vi "ACT_Loop.vi"() -> ()   [LabVIEW 2023, in "Lift_ACT.lvlib"]
uses:
  Lift_ACT.lvlib
  RoboRIO Utilities/Global_STOP.vi
  ENUM_ACT_Action.ctl
  ENUM_ACT_State.ctl
  Global_CMD_ACT_Data In.vi
  Global_ACT_Data Out.vi
  Cluster_CMD_ACT_Data.ctl
  <vilib>/Rock Robotics/WPI/MotorControl/WPI_MotorControlType.ctl
  <vilib>/Rock Robotics/SystemInterfaces/DIO/FPGA_DIOPWMChannel.ctl
  <vilib>/Rock Robotics/WPI/PWM/WPI_PWMDeadband.ctl
  <vilib>/Rock Robotics/SystemInterfaces/DIO/FPGA_DIOChannel.ctl
  <vilib>/Rock Robotics/WPI/MotorControl/WPI_MotorControlDeviceRef.ctl
  <vilib>/Rock Robotics/WPI/ThirdParty/Phoenix-LabVIEW/Motor Controller/Controls/CTRE_Phoenix_MotorControl_TalonFXInvertType.ctl
  <vilib>/Rock Robotics/WPI/ThirdParty/Phoenix-LabVIEW/Motor Controller/Controls/CTRE_Phoenix_MotorControl_NeutralMode.ctl
  Shared Code/TypeDefs/Cluster_FWD  REV Values.ctl
  Shared Code/TypeDefs/Cluster_Config Motor Output.ctl
  Shared Code/TypeDefs/Cluster_PID Gains.ctl
  Shared Code/TypeDefs/Cluster_High-Low.ctl
  Shared Code/TypeDefs/Cluster_PID Config.ctl
  Shared Code/TypeDefs/Cluster_Motion Magic Parameters.ctl
  <vilib>/Rock Robotics/WPI/ThirdParty/Phoenix-LabVIEW/Motor Controller/Controls/CTRE_Phoenix_MotorControl_LimitSwitchNormal.ctl
  Shared Code/TypeDefs/Cluser_Hard Limits.ctl
  Shared Code/TypeDefs/Cluser_Enable-Value I32.ctl
  Shared Code/TypeDefs/Cluser_Config_Soft Limits.ctl
  Shared Code/TypeDefs/Cluser_Limit Travel Config.ctl
  b5508d6c-c1cc-4273-80c5-2077d34e1483.vi
  5f725c2a-0ce1-4524-8967-e83b15fdce90.vi
  <vilib>/Rock Robotics/WPI/ThirdParty/Phoenix-LabVIEW/Motor Controller/Controls/CTRE_Phoenix_MotorControl_ControlMode.ctl
  Shared Code/TypeDefs/Cluster_FX CloseLoop Values.ctl
  Shared Code/TypeDefs/Cluster_FX Limit Switchs.ctl
  Shared Code/TypeDefs/Cluster_FX Current Values.ctl
  Shared Code/TypeDefs/Cluster_Config_Cancoder Data.ctl
  <vilib>/Rock Robotics/WPI/ThirdParty/Phoenix-LabVIEW/CANCoder/Controls/CTRE_Phoenix_CANcoder_DeviceRef.ctl
  Shared Code/TypeDefs/Cluster_FX Sensor Values.ctl
  4f1f8321-3dc8-4b28-8619-20673fc77ec2.vi
  36677ea0-a1a5-47a3-bc56-4475cb7c281e.vi
  573e44c0-11f4-4bd9-ad56-904ec25dba75.vi
  e7494af9-f670-4352-9dfa-ae6ce50709ea.vi
  6201c2b1-dcd8-4430-86f1-9b4ee56c7753.vi
  Shared Code/TypeDefs/Cluster_Lift_Config HW Values.ctl
  Shared Code/TypeDefs/Cluster_Lift_Config SW Values.ctl
  Shared Code/TypeDefs/Cluster_Lift_HW Outputs.ctl
  Shared Code/TypeDefs/Cluster_Lift_SW Output Data.ctl
  5a6858c7-91b3-4b8f-b750-ef97bd4cf642.vi
  89a2f430-b809-46a3-beae-127ce7f74435.vi
  <vilib>/Rock Robotics/WPI/ThirdParty/Phoenix-LabVIEW/CANCoder/Get/CTRE_Phoenix_CANcoder_GetSensorData.vi
  Shared Code/TypeDefs/Cluster_FX Integrated Sensor Values.ctl
  Shared Code/TypeDefs/ENUM_Lift_CMD_Mode Select.ctl
  Shared Code/TypeDefs/Cluser_CAN Follower Data.ctl
  Shared Code/TypeDefs/Cluser_Config_Current Limits.ctl
panel:
  in  "CMD Override":enum32{"None", "Velocity", "Position", "STOP"}(tab)
  in  "Velocity":dbl(slide) scale=-0.2..0.2
  in  "Target Counts":i32
  in  "Positon GO":bool
  out "Current Time":timestamp
  in  "SW Config":T1={"LiftSW Ver"=0, "At Position Delay(S)"=0.2}
  out "SW Output":T2
  in  "Reset zero Offset on Limit Switch":bool
  out "Sensor Read time":dbl format="%.3f"
  out "HW Outputs":T3
  in  "Read Saved Config":bool
  in  "Update Config":bool
  in  "HW Config":T9={"LiftHW Ver"=0, "CAN"={"ID Primary"=0, "Bus"="", "ID Follower"=0}, "Output"={"Type"=enum."Counter-Clockwise", "Neutral"=enum."EEPROMSetting", "Max"={"FWD"=0.0, "REV"=0.0}, "Min"={"FWD"=0.0, "REV"=0.0}, "OL Ramp Rate (S)"=0.0, "Dead Band"=0.0}, "CLUp"={"Gains"={"P"=0.0, "I"=0.0, "D"=0.0, "F"=0.0}, "Error Allowed"={"High"=0.0, "Low"=0.0}, "I Zone"={"High"=0.0, "Low"=0.0}, "Max Out"={"FWD"=0.0, "REV"=0.0}, "Max I Accu"={"High"=0.0, "Low"=0.0}, "CL Ramp Rate (S)"=0.0}, "MM"={"Cruise Velocity"=0, "Acceleration"=0}, "TravelLimits"={"Hard"={"FWD Switch Normal"=enum."Normally Open", "FWD On will Zero Encoder "=FALSE, "REV Switch Normal"=enum."Normally Open", "REV On will Zero Encoder "=FALSE}, "Soft"={"FWD"={"Enable"=FALSE, "Counts"=0}, "REV"={"Enable"=FALSE, "Counts"=0}}}, "Cancoder"={"ID"=0, "CW(t) CCW(f)"=TRUE, "Zero Offset"=0.0}, "CLDown"={"Gains"={"P"=1.0, "I"=0.01, "D"=0.0, "F"=0.0}, "Error Allowed"={"High"=0.0, "Low"=0.0}, "I Zone"={"High"=10000.0, "Low"=-1000.0}, "Max Out"={"FWD"=1.0, "REV"=-1.0}, "Max I Accu"={"High"=10.0, "Low"=-10.0}, "CL Ramp Rate (S)"=0.0}, "CurrentLimit"={"Enable"=FALSE, "Current Limit"=0.0, "Threshold Current"=0.0, "Threshold Time"=0.0}} {"CLDown"."Max I Accu"."Low" format="%#.8f"; "CLDown"."Max I Accu"."High" format="%#.8f"; "CLDown"."Gains"."F" format="%#.8f"; "CLDown"."Gains"."D" format="%#.8f"; "CLDown"."Gains"."I" format="%#.8f"; "CLDown"."Gains"."P" format="%#.8f"; "CLDown"."Error Allowed"."Low" format="%#.8f"; "CLDown"."Error Allowed"."High" format="%#.8f"; "CLDown"."I Zone"."Low" format="%#.8f"; "CLDown"."I Zone"."High" format="%#.8f"; "CLDown"."Max Out"."REV" format="%.2f"; "CLDown"."Max Out"."FWD" format="%.2f"; "TravelLimits"."Soft"."REV"."Counts" format="%#.0f"; "TravelLimits"."Soft"."FWD"."Counts" format="%#.0f"; "Output"."Min"."REV" format="%.2f"; "Output"."Min"."FWD" format="%.2f"; "Output"."Max"."REV" format="%.2f"; "Output"."Max"."FWD" format="%.2f"; "CLUp"."Max I Accu"."Low" format="%#.8f"; "CLUp"."Max I Accu"."High" format="%#.8f"; "CLUp"."Gains"."F" format="%#.8f"; "CLUp"."Gains"."D" format="%#.8f"; "CLUp"."Gains"."I" format="%#.8f"; "CLUp"."Gains"."P" format="%#.8f"; "CLUp"."Error Allowed"."Low" format="%#.8f"; "CLUp"."Error Allowed"."High" format="%#.8f"; "CLUp"."I Zone"."Low" format="%#.8f"; "CLUp"."I Zone"."High" format="%#.8f"; "CLUp"."Max Out"."REV" format="%.2f"; "CLUp"."Max Out"."FWD" format="%.2f"}
  out "CMD":T26
  out "Cycle Time (S)":dbl format="%.3g"
  # "STOP"
  # "Tune Output\nto 1023 Max"
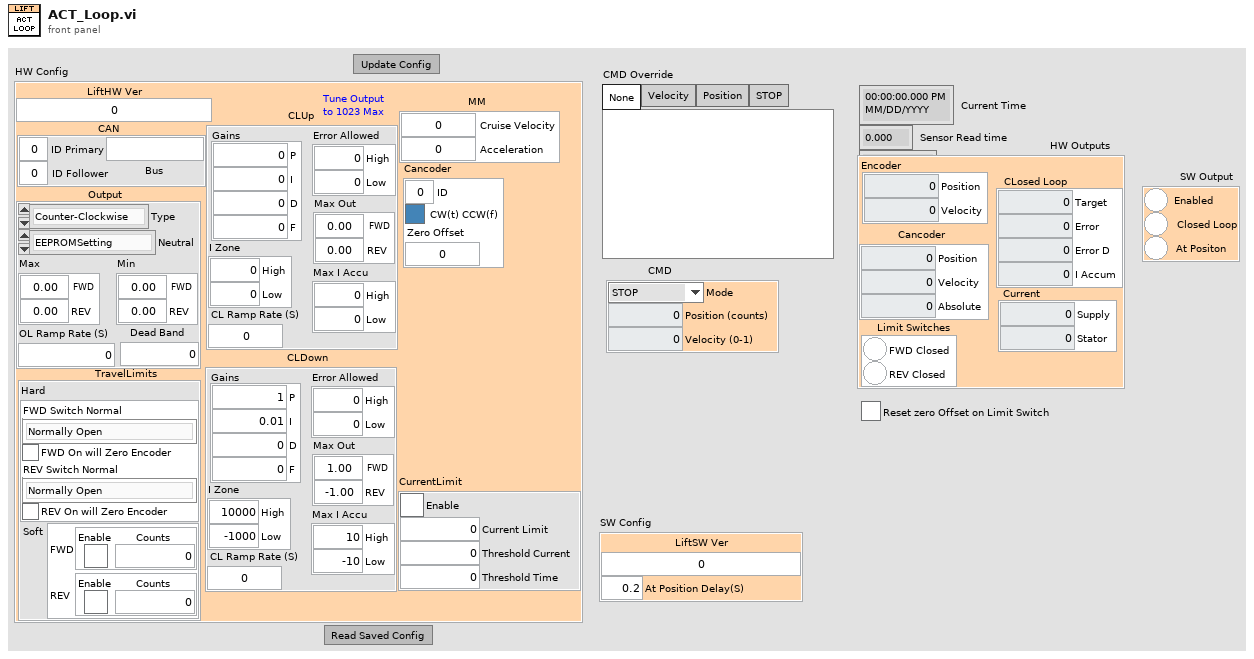
[diagram p1: front panel]
types:
  T1 = typedef "Cluster_Lift_Config SW Values.ctl" = cluster{"LiftSW Ver":u64, "At Position Delay(S)":dbl}
  T2 = typedef "Cluster_Lift_SW Output Data.ctl" = cluster{"Enabled":bool, "Closed Loop":bool, "At Positon":bool}
  T3 = typedef "Cluster_Lift_HW Outputs.ctl" = cluster{"Encoder":T4, "CLosed Loop":T5, "Limit Switches":T6, "Current":T7, "Cancoder":T8}
  T4 = typedef "Cluster_FX Sensor Values.ctl" = cluster{"Position":i32, "Velocity":i32}
  T5 = typedef "Cluster_FX CloseLoop Values.ctl" = cluster{"Target":dbl, "Error":i32, "Error D":dbl, "I Accum":dbl}
  T6 = typedef "Cluster_FX Limit Switchs.ctl" = cluster{"FWD Closed":bool, "REV Closed":bool}
  T7 = typedef "Cluster_FX Current Values.ctl" = cluster{"Supply":dbl, "Stator":dbl}
  T8 = typedef "Cluster_FX Integrated Sensor Values.ctl" = cluster{"Position":dbl, "Velocity":dbl, "Absolute":dbl}
  T9 = typedef "Cluster_Lift_Config HW Values.ctl" = cluster{"LiftHW Ver":u64, "CAN":T10, "Output":T11, "CLUp":T15, "MM":T18, "TravelLimits":T19, "Cancoder":T24, "CLDown":T15, "CurrentLimit":T25}
  T10 = typedef "Cluser_CAN Follower Data.ctl" = cluster{"ID Primary":u8, "Bus":string, "ID Follower":u8}
  T11 = typedef "Cluster_Config Motor Output.ctl" = cluster{"Type":T12, "Neutral":T13, "Max":T14, "Min":T14, "OL Ramp Rate (S)":dbl, "Dead Band":dbl}
  T12 = typedef "CTRE_Phoenix_MotorControl_TalonFXInvertType.ctl" = enum16{"Counter-Clockwise", "Clockwise"}
  T13 = typedef "CTRE_Phoenix_MotorControl_NeutralMode.ctl" = enum8{"EEPROMSetting", "Override to Coast", "Override to Brake"}
  T14 = typedef "Cluster_FWD  REV Values.ctl" = cluster{"FWD":dbl, "REV":dbl}
  T15 = typedef "Cluster_PID Config.ctl" = cluster{"Gains":T16, "Error Allowed":T17, "I Zone":T17, "Max Out":T14, "Max I Accu":T17, "CL Ramp Rate (S)":dbl}
  T16 = typedef "Cluster_PID Gains.ctl" = cluster{"P":dbl, "I":dbl, "D":dbl, "F":dbl}
  T17 = typedef "Cluster_High-Low.ctl" = cluster{"High":dbl, "Low":dbl}
  T18 = typedef "Cluster_Motion Magic Parameters.ctl" = cluster{"Cruise Velocity":i32, "Acceleration":i32}
  T19 = typedef "Cluser_Limit Travel Config.ctl" = cluster{"Hard":T20, "Soft":T22}
  T20 = typedef "Cluser_Hard Limits.ctl" = cluster{"FWD Switch Normal":T21, "FWD On will Zero Encoder ":bool, "REV Switch Normal":T21, "REV On will Zero Encoder ":bool}
  T21 = typedef "CTRE_Phoenix_MotorControl_LimitSwitchNormal.ctl" = enum16{"Normally Open", "Normally Closed", "Disabled"}
  T22 = typedef "Cluser_Config_Soft Limits.ctl" = cluster{"FWD":T23, "REV":T23}
  T23 = typedef "Cluser_Enable-Value I32.ctl" = cluster{"Enable":bool, "Counts":i32}
  T24 = typedef "Cluster_Config_Cancoder Data.ctl" = cluster{"ID":u8, "CW(t) CCW(f)":bool, "Zero Offset":dbl}
  T25 = typedef "Cluser_Config_Current Limits.ctl" = cluster{"Enable":bool, "Current Limit":dbl, "Threshold Current":dbl, "Threshold Time":dbl}
  T26 = typedef "Lift_ACT.lvlib/Cluster_CMD_ACT_Data.ctl" = cluster{"Mode":T27, "Position (counts)":i32, "Velocity (0-1)":dbl}
  T27 = typedef "ENUM_Lift_CMD_Mode Select.ctl" = enum16{"STOP", "Position", "Percent out"}
  T28 = typedef "CTRE_Phoenix_CANcoder_DeviceRef.ctl" = cluster{"DeviceStatus":errorcluster, "Device Number":u8, "Handle":u64, "UsageFrame":u32, "Library Path":path}
  T29 = typedef "CTRE_Phoenix_MotorControl_ControlMode.ctl" = u16
  T30 = typedef "WPI_MotorControlDeviceRef.ctl" = cluster{"DeviceStatus":errorcluster, "Type":T31, "PWM":cluster{"PWM Channel":T32, "DeadBand":T33}, "CAN":cluster{"Device Number":u8, "SetOutput VI Ref":variant, "GetOutput VI Ref":variant, "Enable VI Ref":variant, "Disable VI Ref":variant, "Data":variant}, "Invert":bool, "DIO PWM":cluster{"PWM \"Enable\" Channel":T32, "DIOChannel":T34, "PWM Rate":dbl}}
  T31 = typedef "WPI_MotorControlType.ctl" = enum16{"PWM", "CAN", "DIO PWM"}
  T32 = typedef "FPGA_DIOPWMChannel.ctl" = enum8{"PWM 0", "PWM 1", "PWM 2", "PWM 3", "PWM 4", "PWM 5", "PWM 6", "PWM 7", "PWM 8", "PWM 9", "PWM MXP 0", "PWM MXP 1", "PWM MXP 2", "PWM MXP 3", "PWM MXP 4", "PWM MXP 5", "PWM MXP 6", "PWM MXP 7", "PWM MXP 8", "PWM MXP 9", "Invalid"}
  T33 = typedef "WPI_PWMDeadband.ctl" = cluster{"Name":string, "maxPositivePwm":i32, "minPositivePwm":i32, "centerPwm":i32, "maxNegativePwm":i32, "minNegativePwm":i32, "angularRange":u16}
  T34 = typedef "FPGA_DIOChannel.ctl" = enum8{"DIO 0", "DIO 1", "DIO 2", "DIO 3", "DIO 4", "DIO 5", "DIO 6", "DIO 7", "DIO 8", "DIO 9", "DIO MXP 0", "DIO MXP 1", "DIO MXP 2", "DIO MXP 3", "DIO MXP 4", "DIO MXP 5", "DIO MXP 6", "DIO MXP 7", "DIO MXP 8", "DIO MXP 9", "DIO MXP 10", "DIO MXP 11", "DIO MXP 12", "DIO MXP 13", "DIO MXP 14", "DIO MXP 15", "SPI Port CS1", "SPI Port CS2", "SPI Port CS3", "SPI Port MISO", "SPI Port MOSI", "Invalid"}
  T35 = typedef "Lift_ACT.lvlib/ENUM_ACT_State.ctl" = enum16{"Startup", "Configuring", "Stopping", "Moving Position", "Moving Velocity", "Shutdown"}
  T36 = cluster{"Falcon Ref":T30, "State":T35, "Previous State":T35, "Current Time":timestamp, "Previous Time":timestamp, "Start Time":timestamp, "Target Time (ms)":u32, "Cycle Time(S)":dbl, "ACT Input":T26, "ACT Output DBL":dbl, "Team Files Folder":path, "HW Config":T9, "Update Display":bool, "Max # Of Config Tries":i32, "CAN Timeout":u32, "FX Mode":T29, "FX Set Value":dbl, "HW Outputs":T3, "CANcoder Ref":T28, "SW Outputs":T2, "SW Config":T1}
  T37 = enum16{"FollowerType_PercentOutput", "FollowerType_AuxOutput1"}
  T38 = typedef "Lift_ACT.lvlib/ENUM_ACT_Action.ctl" = enum16{"No Action", "Reset Time", "Reset All", "Config HW File Read", "Config HW File Save", "Config SW File Read", "Config SW File Save", "Config From FP", "Config HW Get", "Config HW Set", "Open HW Only", "Control FX Stop", "Control FX Positon", "Control FX Speed", "Config Cancoder Get Offset Value", "Control FX MotionMagic"}
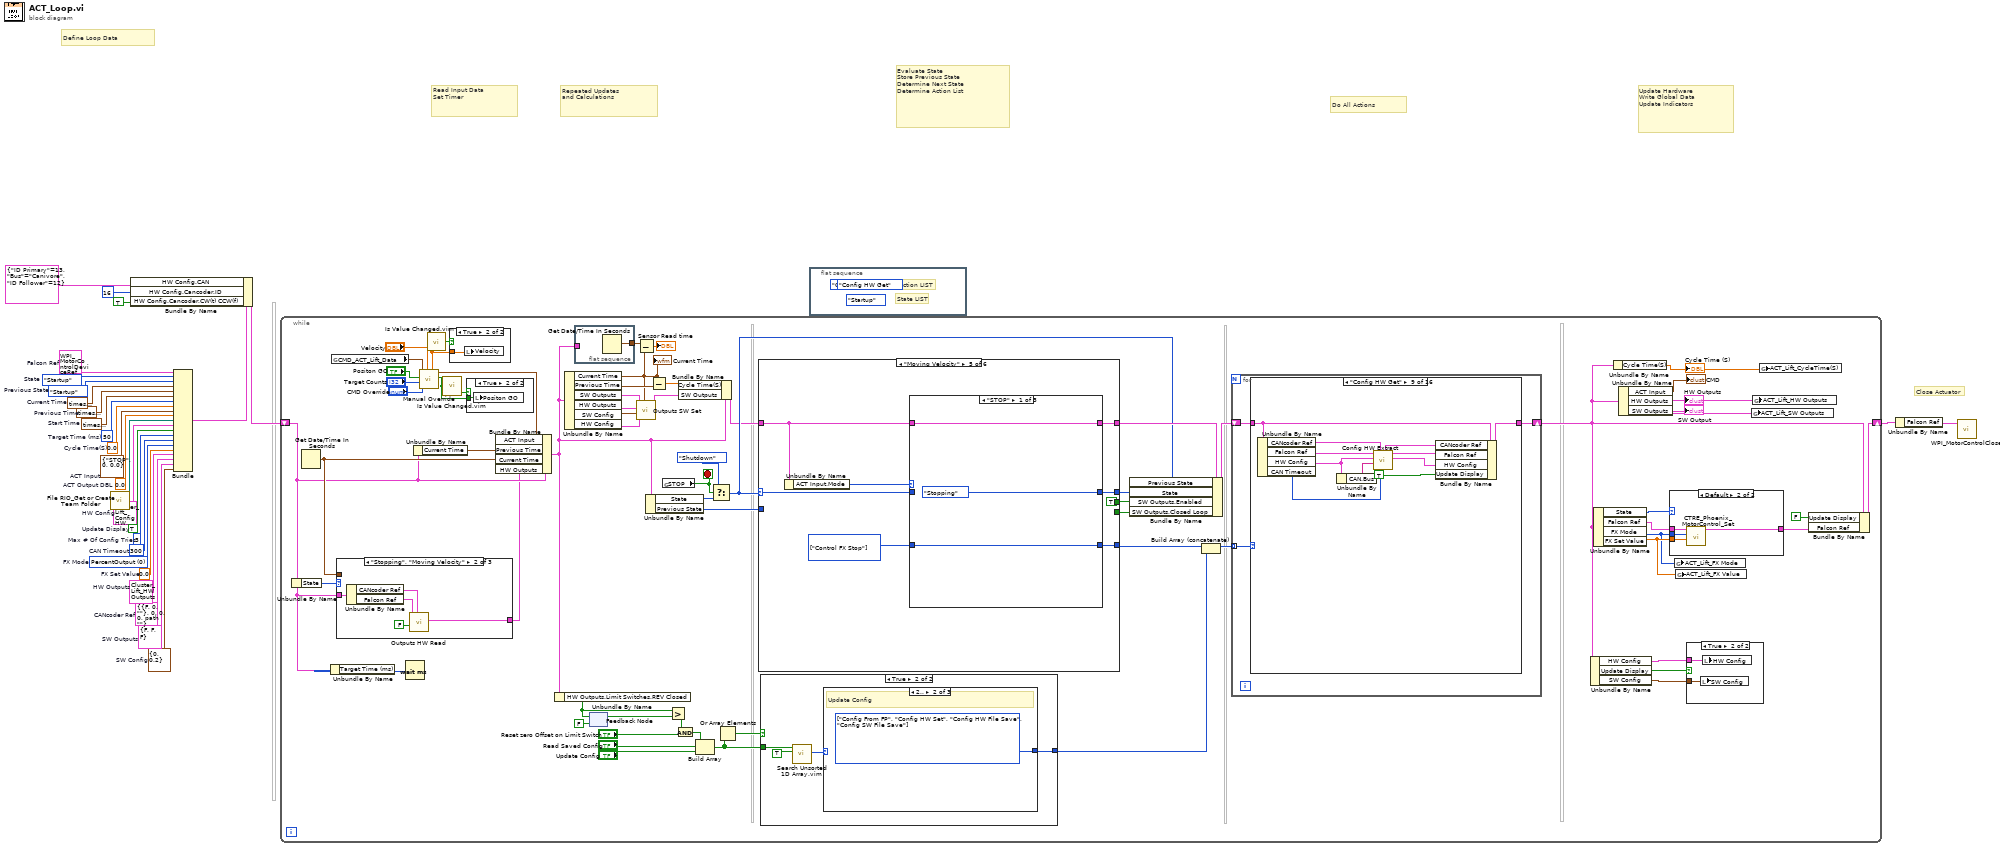
[diagram p0: block diagram]
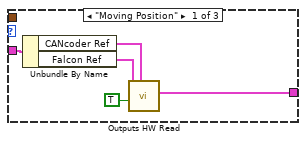
[diagram p4: hidden frame]
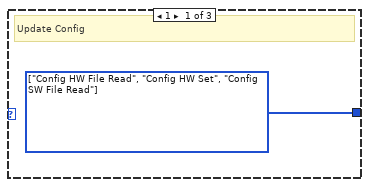
[diagram p7: hidden frame]
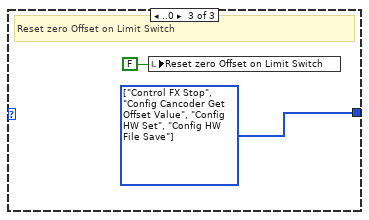
[diagram p8: hidden frame]
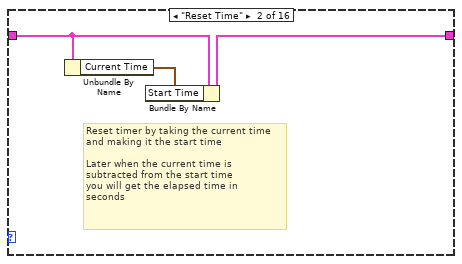
[diagram p12: hidden frame]
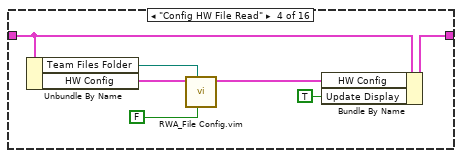
[diagram p14: hidden frame]
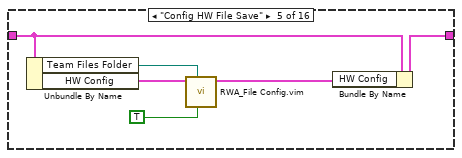
[diagram p15: hidden frame]
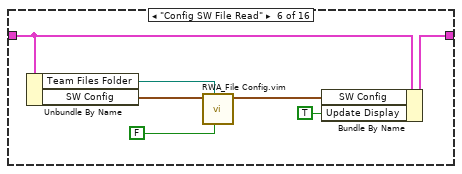
[diagram p16: hidden frame]
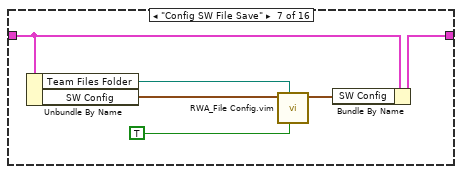
[diagram p17: hidden frame]
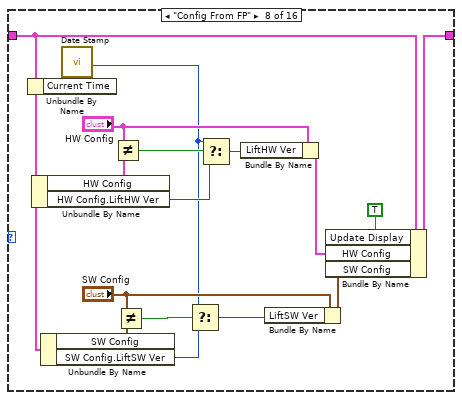
[diagram p18: hidden frame]
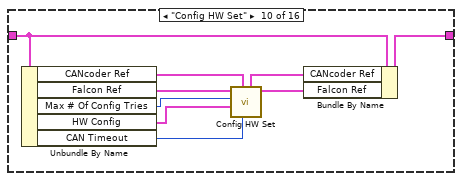
[diagram p19: hidden frame]
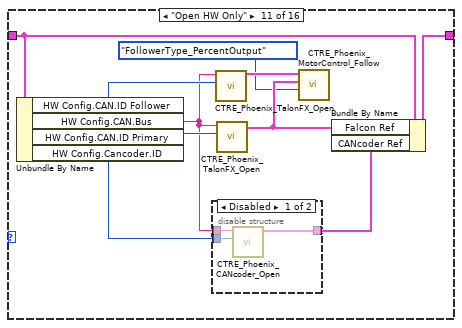
[diagram p20: hidden frame]
diagram:
  w2 = T1 {"LiftSW Ver"=0, "At Position Delay(S)"=0.2}  # SW Config
  w3 = T2 {"Enabled"=FALSE, "Closed Loop"=FALSE, "At Positon"=FALSE}  # SW Outputs
  w6 = T28 {"DeviceStatus"={"status"=FALSE, "code"=0, "source"=""}, "Device Number"=0, "Handle"=0, "UsageFrame"=0, "Library Path"=path ""}  # CANcoder Ref
  w7 = T3 {"Encoder"={"Position"=0, "Velocity"=0}, "CLosed Loop"={"Target"=0.0, "Error"=0, "Error D"=0.0, "I Accum"=0.0}, "Limit Switches"={"FWD Closed"=FALSE, "REV Closed"=FALSE}, "Current"={"Supply"=0.0, "Stator"=0.0}, "Cancoder"={"Position"=0.0, "Velocity"=0.0, "Absolute"=0.0}}  # HW Outputs
  w9 = 0.0  # FX Set Value
  w10 = T29 0 items=["PercentOutput"=0, "Position"=1, "Velocity"=2, "Current"=3, "Follower"=5, "MotionProfile"=6, "MotionMagic"=7, "MotionProfileArc"=10, "Disabled"=15]  # FX Mode
  w11 = u32 300  # CAN Timeout
  w12 = 3  # Max # Of Config Tries
  w13 = TRUE  # Update Display
  w14 = T9 {"LiftHW Ver"=0, "CAN"={"ID Primary"=0, "Bus"="", "ID Follower"=0}, "Output"={"Type"=enum."Counter-Clockwise", "Neutral"=enum."EEPROMSetting", "Max"={"FWD"=0.0, "REV"=0.0}, "Min"={"FWD"=0.0, "REV"=0.0}, "OL Ramp Rate (S)"=0.0, "Dead Band"=0.0}, "CLUp"={"Gains"={"P"=0.0, "I"=0.0, "D"=0.0, "F"=0.0}, "Error Allowed"={"High"=0.0, "Low"=0.0}, "I Zone"={"High"=0.0, "Low"=0.0}, "Max Out"={"FWD"=0.0, "REV"=0.0}, "Max I Accu"={"High"=0.0, "Low"=0.0}, "CL Ramp Rate (S)"=0.0}, "MM"={"Cruise Velocity"=0, "Acceleration"=0}, "TravelLimits"={"Hard"={"FWD Switch Normal"=enum."Normally Open", "FWD On will Zero Encoder "=FALSE, "REV Switch Normal"=enum."Normally Open", "REV On will Zero Encoder "=FALSE}, "Soft"={"FWD"={"Enable"=FALSE, "Counts"=0}, "REV"={"Enable"=FALSE, "Counts"=0}}}, "Cancoder"={"ID"=0, "CW(t) CCW(f)"=FALSE, "Zero Offset"=0.0}, "CLDown"={"Gains"={"P"=1.0, "I"=0.01, "D"=0.0, "F"=0.0}, "Error Allowed"={"High"=0.0, "Low"=0.0}, "I Zone"={"High"=10000.0, "Low"=-1000.0}, "Max Out"={"FWD"=1.0, "REV"=-1.0}, "Max I Accu"={"High"=10.0, "Low"=-10.0}, "CL Ramp Rate (S)"=0.0}, "CurrentLimit"={"Enable"=FALSE, "Current Limit"=0.0, "Threshold Current"=0.0, "Threshold Time"=0.0}}  # HW Config
  w16 = T30 {"DeviceStatus"={"status"=FALSE, "code"=0, "source"=""}, "Type"=enum."PWM", "PWM"={"PWM Channel"=enum."PWM 1", "DeadBand"={"Name"="", "maxPositivePwm"=0, "minPositivePwm"=0, "centerPwm"=0, "maxNegativePwm"=0, "minNegativePwm"=0, "angularRange"=0}}, "CAN"={"Device Number"=0, "SetOutput VI Ref"=variant(enum8{"Percent VBus", "Current", "Speed", "Position", "Voltage"} enum."Percent VBus"), "GetOutput VI Ref"=variant(refnum<k1> refnum), "Enable VI Ref"=variant(dbl 12.0), "Disable VI Ref"=variant(enum8{"Percent VBus", "Speed", "Position", "Slave", "Unchanged / Invalid", "Voltage Compensation", "Current", "Motion Profile"} enum."Percent VBus"), "Data"=variant}, "Invert"=FALSE, "DIO PWM"={"PWM \"Enable\" Channel"=enum."Invalid", "DIOChannel"=enum."Invalid", "PWM Rate"=0.0}}  # Falcon Ref
  w20 = 0.0  # Cycle Time(S)
  w21 = ENUM_ACT_State."Startup"  # Previous State
  w22 = timestamp(0 s since 1904-01-01)  # Previous Time
  w23 = u32 50  # Target Time (ms)
  w24 = 0.0  # ACT Output DBL
  w25 = T26 {"Mode"=enum."STOP", "Position (counts)"=0, "Velocity (0-1)"=0.0}  # ACT Input
  w26 = timestamp(0 s since 1904-01-01)  # Start Time
  w27 = timestamp(0 s since 1904-01-01)  # Current Time
  w28 = ENUM_ACT_State."Startup"  # State
  # "Close Actuator"
  # "Define Loop Data"
  # "Repeated Updates\nand Calculations"
  # "Read Input Data\nSet Timer"
  # "Evaluate State\nStore Previous State\nDetermine Next State\nDetermine Action List"
  # "Do All Actions"
  # "Update Hardware\nWrite Global Data\nUpdate Indicators"
  n1 = call "File RIO_Get or Create Team Folder.vi"() -> ("Team Files Folder"=w15:path)  [unwired: 10 in, 1 out]
  n2 = Bundle("Falcon Ref"=w16, "State"=w28, "Previous State"=w21, "Current Time"=w27, "Previous Time"=w22, "Start Time"=w26, "Target Time (ms)"=w23, "Cycle Time(S)"=w20, "ACT Input"=w25, "ACT Output DBL"=w24, "Team Files Folder"=w15, "HW Config"=w14, "Update Display"=w13, "Max # Of Config Tries"=w12, "CAN Timeout"=w11, "FX Mode"=w10, "FX Set Value"=w9, "HW Outputs"=w7, "CANcoder Ref"=w6, "SW Outputs"=w3, "SW Config"=w2) -> (w18:T36)  [unwired: 1 in]
  n3 = Bundle By Name(cluster=w18, "HW Config.CAN"=T10 {"ID Primary"=13, "Bus"="Canivore", "ID Follower"=12}, "HW Config.Cancoder.ID"=u8 16 ("Wrist Config.Cancoder.ID"), "HW Config.Cancoder.CW(t) CCW(f)"=TRUE ("Wrist Config.Cancoder.CW(t) CCW(f)")) -> (w17:T36)
  n4 = while {
    shift-right: [w77] -> w19
    shift-left: w17 -> [w31]
    stop <- w91 stop-if-true
    n5 = Unbundle By Name(w31) -> ("State"=w67:T35)
    n6 = Get Date/Time In Seconds() -> (seconds since 1Jan1904=w63:timestamp)
    n7 = Unbundle By Name(w31) -> ("Target Time (ms)"=w88:u32)
    n8 = global read "Global_CMD_ACT_Data In.vi" "CMD_ACT_Lift_Data"() -> (w32:T26)
    n9 = case shown="\"Stopping\", \"Moving Velocity\"" w67 {
      tunnel: w31 -> [w102 w107 _]
      tunnel: w63 -> [_ _ _]
      tunnel: [w99 w104 _] -> w29
      frame "Moving Position" {
        n10 = Unbundle By Name(w102) -> ("CANcoder Ref"=w98:T28, "Falcon Ref"=w101:T30)
        n11 = call "Outputs HW Read.vi"("CTRE_CANcoder_DeviceRef"=w98, "Read Closed Loop"=TRUE, "Ref"=w101) -> ("Sensor Values Out"=w99:T3)  [unwired: 5 in, 3 out]
      }
      frame "Stopping", "Moving Velocity" {
        n12 = Unbundle By Name(w107) -> ("CANcoder Ref"=w103:T28, "Falcon Ref"=w106:T30)
        n13 = call "Outputs HW Read.vi"("CTRE_CANcoder_DeviceRef"=w103, "Read Closed Loop"=FALSE, "Ref"=w106) -> ("Sensor Values Out"=w104:T3)  [unwired: 5 in, 3 out]
      }
      frame "Startup", "Configuring", "Shutdown" {
      }
    }
    n14 = Wait (ms)(milliseconds to wait=w88) -> ()  [unwired: 1 out]
    n15 = Unbundle By Name(w31) -> ("Current Time"=w87:timestamp)
    n16 = call "Manual Override.vi"("Velocity"="Velocity", "Override"="CMD Override", "Counts"="Target Counts", "Position GO"="Positon GO", "Auto CMD"=w32) -> ("Position GO Out"=w40:bool, "OverRide Command Out"=w33:T26, "Velocity Out"=w38:dbl)  [unwired: 4 in]
    n17 = call "Is Value Changed.vim"("value"=w38) -> ("changed or first call?"=w39:bool)
    n18 = call "Is Value Changed.vim"("value"=w40) -> ("changed or first call?"=w41:bool)
    n19 = case shown="True" w39 {
      tunnel: w38 -> [_ w96]
      frame False {
      }
      frame True {
        n20 = local write "Velocity"(w96) -> ()
      }
    }
    n21 = case shown="True" w41 {
      tunnel: w40 -> [_ w95]
      frame False {
      }
      frame True {
        n22 = local write "Positon GO"(w95) -> ()
      }
    }
    n23 = Bundle By Name(cluster=w31, "ACT Input"=w33, "Previous Time"=w87, "Current Time"=w63, "HW Outputs"=w29) -> (w30:T36)
    n24 = Unbundle By Name(w30) -> ("HW Outputs.Limit Switches.REV Closed"=w56:bool)
    n25 = Unbundle By Name(w30) -> ("Current Time"=w45:timestamp, "Previous Time"=w84:timestamp, "SW Outputs"=w48:T2, "HW Outputs"=w46:T3, "SW Config"=w44:T1, "HW Config"=w43:T9)
    "Current Time" <- w45
    n26 = flat-sequence {
      tunnel: [w97] -> w65
      tunnel: w30 -> [_]
      frame #0 {
        n27 = Get Date/Time In Seconds() -> (seconds since 1Jan1904=w97:timestamp)
      }
    }
    n28 = feedback #1(FALSE ("REV Closed")) -> (w57:bool)
    n29 = feedback-in #1(w56) -> ()
    n30 = call "Outputs SW Set.vi"("Current Time"=w45, "HW Config"=w43, "SW Config"=w44, "Outputs FX"=w46, "SW Output"=w48) -> ("SW Output Out"=w47:T2)  [unwired: 6 in]
    n31 = Subtract(x=w65, y=w45) -> (x-y=→"Sensor Read time":dbl)
    n32 = Unbundle By Name(w30) -> ("State"=w89:T35, "Previous State"=w86:T35)
    n33 = Subtract(x=w45, y=w84) -> (x-y=w82:dbl)
    n34 = global read "Global_STOP.vi" "STOP"() -> (w91:bool)
    n35 = Greater?(x=w56, y=w57) -> (0:w54:bool)
    n36 = And(x=w54, y="Reset zero Offset on Limit Switch") -> (x .and. y?=w53:bool)
    n37 = Bundle By Name(cluster=w30, "Cycle Time(S)"=w82, "SW Outputs"=w47) -> (w83:T36)
    n38 = Build Array(w53, "Read Saved Config", "Update Config") -> (w59:bool[])
    n39 = Select(t=ENUM_ACT_State."Shutdown" ("State"), s=w91, f=w89) -> (s? t:f=w85:T35)
    n40 = Or Array Elements(Boolean array=w59) -> (logical OR=w60:bool)
    n41 = case shown="\"Moving Velocity\"" w85 {
      selector: w85 -> [_ _ _ w276 w293 _]
      tunnel: w83 -> [w232 w238 w262 w277 w294 w309]
      tunnel: [w232 w241 w261 w278 w295 w309] -> w93
      tunnel: [ENUM_ACT_State."Configuring" ("State") w240 w260 w280 w297 ENUM_ACT_State."Shutdown" ("State")] -> w92
      tunnel: [w231 w239 w258 w275 w291 w307] -> w81
      tunnel: w86 -> [_ _ _ _ _ _]
      tunnel: [_ _ TRUE w273 TRUE _] -> w50
      tunnel: [_ _ _ w273 _ _] -> w49
      frame "Startup" {
        w231 = T38[] [enum."Reset Time"] items=["No Action", "Reset Time", "Reset All", "Config HW File Read", "Config HW File Save", "Config SW File Read", "Config SW File Save", "Config From FP", "Config HW Get", "Config HW Set", "Open HW Only", "Control FX Stop", "Control FX Positon", "Control FX Speed", "Config Cancoder Get Offset Value", "Control FX MotionMagic"] ("Actions")
      }
      frame "Configuring" {
        n42 = Unbundle By Name(w238) -> ("SW Config"=w236:T1)
        n43 = Unbundle By Name(w238) -> ("Team Files Folder"=w235:path, "HW Config"=w243:T9)
        n44 = call "Config_Build Name.vim"("Config First Name"=w243) -> ("Cfg file"=w245:string)  [unwired: 9 in, 1 out]
        n45 = call "Config_Build Name.vim"("Config First Name"=w236) -> ("Cfg file"=w237:string)  [unwired: 9 in, 1 out]
        n46 = Build Path(base path=w235, name or relative path=w237) -> (appended path=w234:path)
        n47 = Build Path(base path=w235, name or relative path=w245) -> (appended path=w244:path)
        n48 = call <vilib>:"Check if File or Folder Exists.vi"("path"=w234) -> ("file or folder exists?"=w233:bool)  [unwired: 8 in, 2 out]
        n49 = call <vilib>:"Check if File or Folder Exists.vi"("path"=w244) -> ("file or folder exists?"=w242:bool)  [unwired: 8 in, 2 out]
        n50 = case shown="True" w242 {
          tunnel: w238 -> [w248 w252]
          tunnel: [w248 w252] -> w241
          tunnel: [ENUM_ACT_State."Configuring" ("State") w251] -> w240
          tunnel: [w246 w250] -> w239
          tunnel: w233 -> [_ w249]
          frame False {
            w246 = T38[] [enum."Open HW Only", enum."Config HW Get", enum."Config HW File Save"] items=["No Action", "Reset Time", "Reset All", "Config HW File Read", "Config HW File Save", "Config SW File Read", "Config SW File Save", "Config From FP", "Config HW Get", "Config HW Set", "Open HW Only", "Control FX Stop", "Control FX Positon", "Control FX Speed", "Config Cancoder Get Offset Value", "Control FX MotionMagic"] ("Actions")
            # "HW Config File Not Found"
          }
          frame True {
            # "HW Config File Found"
            n51 = case shown="False" w249 {
              tunnel: [ENUM_ACT_State."Configuring" ("State") ENUM_ACT_State."Stopping" ("State")] -> w251
              tunnel: [w253 w255] -> w250
              frame False {
                w253 = T38[] [enum."Config SW File Save"] items=["No Action", "Reset Time", "Reset All", "Config HW File Read", "Config HW File Save", "Config SW File Read", "Config SW File Save", "Config From FP", "Config HW Get", "Config HW Set", "Open HW Only", "Control FX Stop", "Control FX Positon", "Control FX Speed", "Config Cancoder Get Offset Value", "Control FX MotionMagic"] ("Actions")
                # "SW Config File NOT Found"
              }
              frame True {
                w255 = T38[] [enum."Config HW File Read", enum."Config HW Set", enum."Config SW File Read", enum."Reset All", enum."Control FX Stop"] items=["No Action", "Reset Time", "Reset All", "Config HW File Read", "Config HW File Save", "Config SW File Read", "Config SW File Save", "Config From FP", "Config HW Get", "Config HW Set", "Open HW Only", "Control FX Stop", "Control FX Positon", "Control FX Speed", "Config Cancoder Get Offset Value", "Control FX MotionMagic"] ("Actions")
                # "SW Config File Found"
              }
            }
          }
        }
      }
      frame "Stopping" {
        w259 = T38[] [enum."Control FX Stop"] items=["No Action", "Reset Time", "Reset All", "Config HW File Read", "Config HW File Save", "Config SW File Read", "Config SW File Save", "Config From FP", "Config HW Get", "Config HW Set", "Open HW Only", "Control FX Stop", "Control FX Positon", "Control FX Speed", "Config Cancoder Get Offset Value", "Control FX MotionMagic"] ("Actions")
        n52 = Unbundle By Name(w262) -> ("ACT Input.Mode"=w263:T27)
        n53 = case shown="\"Percent out\"" w263 {
          tunnel: w262 -> [w266 w269 w272]
          tunnel: [w266 w269 w272] -> w261
          tunnel: [ENUM_ACT_State."Stopping" ("State") ENUM_ACT_State."Moving Position" ("State") ENUM_ACT_State."Moving Velocity" ("State")] -> w260
          tunnel: [w264 w267 w270] -> w258
          tunnel: w259 -> [w264 w267 w270]
          frame "STOP" {
          }
          frame "Position" {
          }
          frame "Percent out" {
          }
        }
      }
      frame "Moving Position" {
        w273 = TRUE
        w274 = T38[] [enum."Control FX Stop"] items=["No Action", "Reset Time", "Reset All", "Config HW File Read", "Config HW File Save", "Config SW File Read", "Config SW File Save", "Config From FP", "Config HW Get", "Config HW Set", "Open HW Only", "Control FX Stop", "Control FX Positon", "Control FX Speed", "Config Cancoder Get Offset Value", "Control FX MotionMagic"] ("Actions")
        n54 = Unbundle By Name(w277) -> ("ACT Input.Mode"=w279:T27)
        n55 = case shown="\"Position\"" w279 {
          tunnel: [ENUM_ACT_State."Stopping" ("State") ENUM_ACT_State."Moving Velocity" ("State") w288] -> w280
          tunnel: w277 -> [w283 w286 w289]
          tunnel: [w283 w286 w289] -> w278
          tunnel: w276 -> [_ _ w288]
          tunnel: [w281 w284 w287] -> w275
          tunnel: w274 -> [w281 w284 _]
          frame "STOP" {
          }
          frame "Percent out" {
          }
          frame "Position" {
            w287 = T38[] [enum."Control FX Positon"] items=["No Action", "Reset Time", "Reset All", "Config HW File Read", "Config HW File Save", "Config SW File Read", "Config SW File Save", "Config From FP", "Config HW Get", "Config HW Set", "Open HW Only", "Control FX Stop", "Control FX Positon", "Control FX Speed", "Config Cancoder Get Offset Value", "Control FX MotionMagic"] ("Actions")
          }
        }
      }
      frame "Moving Velocity" {
        w292 = T38[] [enum."Control FX Stop"] items=["No Action", "Reset Time", "Reset All", "Config HW File Read", "Config HW File Save", "Config SW File Read", "Config SW File Save", "Config From FP", "Config HW Get", "Config HW Set", "Open HW Only", "Control FX Stop", "Control FX Positon", "Control FX Speed", "Config Cancoder Get Offset Value", "Control FX MotionMagic"] ("Actions")
        n56 = Unbundle By Name(w294) -> ("ACT Input.Mode"=w296:T27)
        n57 = case shown="\"STOP\"" w296 {
          tunnel: [ENUM_ACT_State."Stopping" ("State") w301 ENUM_ACT_State."Moving Position" ("State")] -> w297
          tunnel: w294 -> [w300 w303 w306]
          tunnel: [w300 w303 w306] -> w295
          tunnel: w293 -> [_ w301 _]
          tunnel: [w298 w302 w304] -> w291
          tunnel: w292 -> [w298 _ w304]
          frame "STOP" {
          }
          frame "Percent out" {
            w302 = T38[] [enum."Control FX Speed"] items=["No Action", "Reset Time", "Reset All", "Config HW File Read", "Config HW File Save", "Config SW File Read", "Config SW File Save", "Config From FP", "Config HW Get", "Config HW Set", "Open HW Only", "Control FX Stop", "Control FX Positon", "Control FX Speed", "Config Cancoder Get Offset Value", "Control FX MotionMagic"] ("Actions")
          }
          frame "Position" {
          }
        }
      }
      frame "Shutdown" {
        w307 = T38[] [enum."Reset All"] items=["No Action", "Reset Time", "Reset All", "Config HW File Read", "Config HW File Save", "Config SW File Read", "Config SW File Save", "Config From FP", "Config HW Get", "Config HW Set", "Open HW Only", "Control FX Stop", "Control FX Positon", "Control FX Speed", "Config Cancoder Get Offset Value", "Control FX MotionMagic"] ("Actions")
      }
    }
    n58 = case shown="True" w60 {
      tunnel: w59 -> [_ w110]
      tunnel: [_ w108] -> w58
      frame False {
      }
      frame True {
        n59 = call "Search Unsorted 1D Array.vim"("element"=TRUE, "unsorted 1D array"=w110) -> ("index of element"=w109:i32)  [unwired: 9 in]
        n60 = case shown="2.." w109 {
          tunnel: [w112 w113 w115] -> w108
          frame 1 {
            w112 = T38[] [enum."Config HW File Read", enum."Config HW Set", enum."Config SW File Read"] items=["No Action", "Reset Time", "Reset All", "Config HW File Read", "Config HW File Save", "Config SW File Read", "Config SW File Save", "Config From FP", "Config HW Get", "Config HW Set", "Open HW Only", "Control FX Stop", "Control FX Positon", "Control FX Speed", "Config Cancoder Get Offset Value", "Control FX MotionMagic"] ("Actions")
            # "Update Config"
          }
          frame 2.. {
            w113 = T38[] [enum."Config From FP", enum."Config HW Set", enum."Config HW File Save", enum."Config SW File Save"] items=["No Action", "Reset Time", "Reset All", "Config HW File Read", "Config HW File Save", "Config SW File Read", "Config SW File Save", "Config From FP", "Config HW Get", "Config HW Set", "Open HW Only", "Control FX Stop", "Control FX Positon", "Control FX Speed", "Config Cancoder Get Offset Value", "Control FX MotionMagic"] ("Actions")
            # "Update Config"
          }
          frame ..0 {
            w115 = T38[] [enum."Control FX Stop", enum."Config Cancoder Get Offset Value", enum."Config HW Set", enum."Config HW File Save"] items=["No Action", "Reset Time", "Reset All", "Config HW File Read", "Config HW File Save", "Config SW File Read", "Config SW File Save", "Config From FP", "Config HW Get", "Config HW Set", "Open HW Only", "Control FX Stop", "Control FX Positon", "Control FX Speed", "Config Cancoder Get Offset Value", "Control FX MotionMagic"] ("Actions")
            # "Reset zero Offset on Limit Switch"
            n61 = local write "Reset zero Offset on Limit Switch"(FALSE ("Reset zero Offset on Limit Switch")) -> ()
          }
        }
      }
    }
    n62 = Bundle By Name(cluster=w93, "Previous State"=w85, "State"=w92, "SW Outputs.Enabled"=w50, "SW Outputs.Closed Loop"=w49) -> (w94:T36)
    n63 = Build Array (concatenate)(w81, w58) -> (w75:T38[])
    n64 = for {
      tunnel: w75 -> [w125] mode=indexing
      shift-right: [w124] -> w74
      shift-left: w94 -> [w123]
      n65 = case shown="\"Config HW Get\"" w125 {
        tunnel: w123 -> [w126 w129 w130 w136 w142 w149 w155 w163 w180 w191 w201 w209 w212 w217 w222 w227]
        tunnel: [w126 w128 w130 w137 w143 w150 w156 w173 w181 w192 w202 w210 w214 w219 w224 w228] -> w124
        frame "No Action" {
        }
        frame "Reset Time" {
          # "Reset timer by taking the current time\nand making it the start time\n\nLater when the current time is \nsubtracted from the start time\nyou will get the elapsed time in \nseconds"
          n66 = Unbundle By Name(w129) -> ("Current Time"=w127:timestamp)
          n67 = Bundle By Name(cluster=w129, "Start Time"=w127) -> (w128:T36)
        }
        frame "Reset All" {
        }
        frame "Config HW File Read" {
          n68 = Unbundle By Name(w136) -> ("Team Files Folder"=w133:path, "HW Config"=w135:T9)
          n69 = call "RWA_File Config.vim"("Read(f) Save(t)"=FALSE ("Read(f) Write(t)"), "Target Folder Folder"=w133, "Any Config"=w135) -> ("Any Config Out"=w134:T9)  [unwired: 4 in, 4 out]
          n70 = Bundle By Name(cluster=w136, "HW Config"=w134, "Update Display"=TRUE) -> (w137:T36)
        }
        frame "Config HW File Save" {
          n71 = Unbundle By Name(w142) -> ("Team Files Folder"=w139:path, "HW Config"=w141:T9)
          n72 = call "RWA_File Config.vim"("Read(f) Save(t)"=TRUE ("Read(f) Write(t)"), "Target Folder Folder"=w139, "Any Config"=w141) -> ("Any Config Out"=w140:T9)  [unwired: 4 in, 4 out]
          n73 = Bundle By Name(cluster=w142, "HW Config"=w140) -> (w143:T36)
        }
        frame "Config SW File Read" {
          n74 = Unbundle By Name(w149) -> ("Team Files Folder"=w146:path, "SW Config"=w148:T1)
          n75 = call "RWA_File Config.vim"("Read(f) Save(t)"=FALSE ("Read(f) Write(t)"), "Target Folder Folder"=w146, "Any Config"=w148) -> ("Any Config Out"=w147:T1)  [unwired: 4 in, 4 out]
          n76 = Bundle By Name(cluster=w149, "SW Config"=w147, "Update Display"=TRUE) -> (w150:T36)
        }
        frame "Config SW File Save" {
          n77 = Unbundle By Name(w155) -> ("Team Files Folder"=w152:path, "SW Config"=w154:T1)
          n78 = call "RWA_File Config.vim"("Read(f) Save(t)"=TRUE ("Read(f) Write(t)"), "Target Folder Folder"=w152, "Any Config"=w154) -> ("Any Config Out"=w153:T1)  [unwired: 4 in, 4 out]
          n79 = Bundle By Name(cluster=w155, "SW Config"=w153) -> (w156:T36)
        }
        frame "Config From FP" {
          n80 = Unbundle By Name(w163) -> ("Current Time"=w172:timestamp)
          n81 = Unbundle By Name(w163) -> ("HW Config"=w162:T9, "HW Config.LiftHW Ver"=w159:u64)
          n82 = Unbundle By Name(w163) -> ("SW Config"=w165:T1, "SW Config.LiftSW Ver"=w167:u64)
          n83 = call "Date Stamp.vi"("Time"=w172) -> ("U64 Out"=w158:u64)  [unwired: 5 in, 1 out]
          n84 = Not Equal?(x="HW Config", y=w162) -> (x != y?=w160:bool)
          n85 = Not Equal?(x=w165, y="SW Config") -> (x != y?=w168:bool)
          n86 = Select(t=w158, s=w168, f=w167) -> (s? t:f=w166:u64)
          n87 = Select(t=w158, s=w160, f=w159) -> (s? t:f=w157:u64)
          n88 = Bundle By Name(cluster="HW Config", "LiftHW Ver"=w157) -> (w171:T9)
          n89 = Bundle By Name(cluster="SW Config", "LiftSW Ver"=w166) -> (w170:T1)
          n90 = Bundle By Name(cluster=w163, "Update Display"=TRUE, "HW Config"=w171, "SW Config"=w170) -> (w173:T36)
        }
        frame "Config HW Get" {
          n91 = Unbundle By Name(w180) -> ("CANcoder Ref"=w175:T28, "Falcon Ref"=w184:T30, "HW Config"=w183:T9, "CAN Timeout"=w176:u32)
          n92 = Unbundle By Name(w183) -> ("CAN.Bus"=w182:string)
          n93 = call "Config HW Extract.vi"("Send Cmd Timout(ms)"=w176, "CANcoderRef"=w175, "CAN.Bus"=w182, "HW Config"=w183, "DevRef"=w184) -> ("HW Config Data Out"=w178:T9, "DevRef Out"=w179:T30, "CANcoderRef Out"=w174:T28)  [unwired: 3 in, 1 out]
          n94 = Bundle By Name(cluster=w180, "CANcoder Ref"=w174, "Falcon Ref"=w179, "HW Config"=w178, "Update Display"=TRUE) -> (w181:T36)
        }
        frame "Config HW Set" {
          n95 = Unbundle By Name(w191) -> ("CANcoder Ref"=w186:T28, "Falcon Ref"=w193:T30, "Max # Of Config Tries"=w187:i32, "HW Config"=w189:T9, "CAN Timeout"=w188:u32)
          n96 = call "Config HW Set.vi"("Send Cmd Timout(ms)"=w188, "CANcoder Ref"=w186, "HW Config"=w189, "Max # Of Tries"=w187, "DevRef"=w193) -> ("DevRef Out Out"=w190:T30, "CANcoder Ref Out"=w185:T28)  [unwired: 4 in, 1 out]
          n97 = Bundle By Name(cluster=w191, "CANcoder Ref"=w185, "Falcon Ref"=w190) -> (w192:T36)
        }
        frame "Open HW Only" {
          n98 = Unbundle By Name(w201) -> ("HW Config.CAN.ID Follower"=w198:u8, "HW Config.CAN.Bus"=w197:string, "HW Config.CAN.ID Primary"=w203:u8, "HW Config.Cancoder.ID"=w200:u8)
          n99 = disable-structure shown="Disabled" {
            disable-tunnel: w197 -> [w206 _]
            disable-tunnel: w200 -> [w205 _]
            disable-tunnel: [w204 _] -> w199
            frame Disabled {
              n100 = call <vilib>:"CTRE_Phoenix_CANcoder_Open.vi"("Device Number"=w205, "CAN Bus"=w206) -> ("CTRE_CANcoder_DeviceRef"=w204:T28)  [unwired: 8 in, 1 out]
            }
            frame Enabled {
            }
          }
          n101 = call <vilib>:"CTRE_Phoenix_TalonFX_Open.vi"("Device Number"=w198, "CAN Bus"=w197) -> ("PhoenixMotorControlDevRef"=w196:T30)  [unwired: 8 in, 1 out]
          n102 = call <vilib>:"CTRE_Phoenix_TalonFX_Open.vi"("Device Number"=w203, "CAN Bus"=w197) -> ("PhoenixMotorControlDevRef"=w195:T30)  [unwired: 8 in, 1 out]
          n103 = call <vilib>:"CTRE_Phoenix_MotorControl_Follow.vi"("FollowerType"=T37."FollowerType_PercentOutput", "Master Controller to Follow"=w195, "PhoenixMotorControlDevRef"=w196) -> ()  [unwired: 7 in, 2 out]
          n104 = Bundle By Name(cluster=w201, "Falcon Ref"=w195, "CANcoder Ref"=w199) -> (w202:T36)
        }
        frame "Control FX Stop" {
          w208 = T29 0 items=["PercentOutput"=0, "Position"=1, "Velocity"=2, "Current"=3, "Follower"=5, "MotionProfile"=6, "MotionMagic"=7, "MotionProfileArc"=10, "Disabled"=15] ("FX Mode")
          n105 = Bundle By Name(cluster=w209, "FX Mode"=w208, "FX Set Value"=0.0) -> (w210:T36)
        }
        frame "Control FX Speed" {
          w213 = T29 0 items=["PercentOutput"=0, "Position"=1, "Velocity"=2, "Current"=3, "Follower"=5, "MotionProfile"=6, "MotionMagic"=7, "MotionProfileArc"=10, "Disabled"=15] ("FX Mode")
          n106 = Unbundle By Name(w212) -> ("ACT Input.Velocity (0-1)"=w211:dbl)
          n107 = Bundle By Name(cluster=w212, "FX Mode"=w213, "FX Set Value"=w211) -> (w214:T36)
        }
        frame "Control FX Positon" {
          w218 = T29 1 items=["PercentOutput"=0, "Position"=1, "Velocity"=2, "Current"=3, "Follower"=5, "MotionProfile"=6, "MotionMagic"=7, "MotionProfileArc"=10, "Disabled"=15] ("FX Mode")
          n108 = Unbundle By Name(w217) -> ("ACT Input.Position (counts)"=w215:i32)
          n109 = To Double Precision Float(number=w215) -> (double precision float=w216:dbl)
          n110 = Bundle By Name(cluster=w217, "FX Mode"=w218, "FX Set Value"=w216) -> (w219:T36)
        }
        frame "Control FX MotionMagic" {
          w223 = T29 7 items=["PercentOutput"=0, "Position"=1, "Velocity"=2, "Current"=3, "Follower"=5, "MotionProfile"=6, "MotionMagic"=7, "MotionProfileArc"=10, "Disabled"=15] ("FX Mode")
          n111 = Unbundle By Name(w222) -> ("ACT Input.Position (counts)"=w220:i32)
          n112 = To Double Precision Float(number=w220) -> (double precision float=w221:dbl)
          n113 = Bundle By Name(cluster=w222, "FX Mode"=w223, "FX Set Value"=w221) -> (w224:T36)
        }
        frame "Config Cancoder Get Offset Value" {
          n114 = Unbundle By Name(w227) -> ("CANcoder Ref"=w229:T28)
          n115 = call-poly <vilib>:"CTRE_Phoenix_CANcoder_GetPolymorphic.vi"("CTRE_CANcoder_DeviceRef"=w229) -> ("Absolute Position"=w226:dbl)  [unwired: 10 in, 4 out]
          n116 = Bundle By Name(cluster=w227, "HW Config.Cancoder.Zero Offset"=w226, "Update Display"=TRUE) -> (w228:T36)
        }
      }
    }
    n117 = Unbundle By Name(w74) -> ("HW Config"=w71:T9, "Update Display"=w72:bool, "SW Config"=w42:T1)
    n118 = Unbundle By Name(w74) -> ("State"=w68:T35, "Falcon Ref"=w79:T30, "FX Mode"=w69:T29, "FX Set Value"=w70:dbl)
    n119 = Unbundle By Name(w74) -> ("Cycle Time(S)"=w76:dbl)
    "Cycle Time (S)" <- w76
    n120 = Unbundle By Name(w74) -> ("ACT Input"=→"CMD":T26, "HW Outputs"=w66:T3, "SW Outputs"=w51:T2)
    "HW Outputs" <- w66
    "SW Output" <- w51
    n121 = case shown="Default" w68 {
      tunnel: w79 -> [w116 w120]
      tunnel: [w116 w119] -> w78
      tunnel: w70 -> [_ w118]
      tunnel: w69 -> [_ w117]
      frame "Startup", "Configuring" {
      }
      frame Default {
        n122 = call <vilib>:"CTRE_Phoenix_MotorControl_Set.vi"("Output"=w118, "Control Mode"=w117, "PhoenixMotorControlDevRef"=w120) -> ("PhoenixMotorControlDevRef"=w119:T30)  [unwired: 7 in, 1 out]
      }
    }
    n123 = global write "Global_ACT_Data Out.vi" "ACT_Lift_FX Mode"(w69) -> ()
    n124 = global write "Global_ACT_Data Out.vi" "ACT_Lift_FX Value"(w70) -> ()
    n125 = case shown="True" w72 {
      tunnel: w71 -> [_ w122]
      tunnel: w42 -> [_ w121]
      frame False {
      }
      frame True {
        n126 = local write "SW Config"(w121) -> ()
        n127 = local write "HW Config"(w122) -> ()
      }
    }
    n128 = global write "Global_ACT_Data Out.vi" "ACT_Lift_SW Outputs"(w51) -> ()
    n129 = global write "Global_ACT_Data Out.vi" "ACT_Lift_HW Outputs"(w66) -> ()
    n130 = global write "Global_ACT_Data Out.vi" "ACT_Lift_CycleTime(S)"(w76) -> ()
    n131 = Bundle By Name(cluster=w74, "Update Display"=FALSE, "Falcon Ref"=w78) -> (w77:T36)
  }
  n132 = flat-sequence {
    frame #0 {
      (unwired) ENUM_ACT_Action."Open HW Only" ("Action")
      (unwired) ENUM_ACT_State."Startup" ("State")
      (unwired) ENUM_ACT_Action."Config HW Get" ("Action")
      # "State LIST"
      # "Action LIST"
    }
  }
  n133 = Unbundle By Name(w19) -> ("Falcon Ref"=w8:T30)
  n134 = call <vilib>:"WPI_MotorControlClose.vi"("MotorControlDevRef"=w8) -> ()  [unwired: 10 in, 1 out]
